vi "Reset.vi"(8 "error in (no error)":errorcluster, 11 "ChromaPowerSupply in":refnum<class "ChromaPowerSupply.lvclass">) -> (0 "error out":errorcluster, 3 "ChromaPowerSupply out":refnum<class "ChromaPowerSupply.lvclass">)   [LabVIEW 2018, in "AcPwrPlugins.lvlib" / "ChromaPowerSupply.lvclass"]
doc: "This VI resets the instrument(s) into a know state."
uses:
  ChromaPowerSupply.lvclass
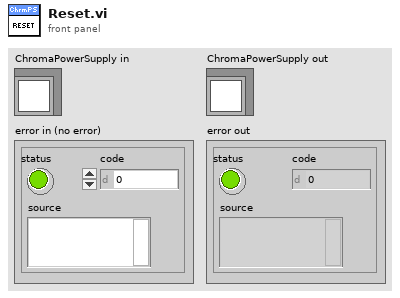
[diagram p1: front panel]
types:
  T1 = typedef "AcPwrPlugins.lvlib/ChromaPowerSupply.lvclass/Device(s)Settings.ctl" = cluster{"Phases":cluster{"Handle":string, "Instrument Options":string, "id query (T)":bool, "reset device (T)":bool, "Timing":cluster{"TimingOn":enum16{""}, "Hours":u32, "Minutes":u32, "Seconds":dbl, "CutoffVoltage":dbl}, "Connected":bool, "Output Mode":enum16{"Voltage (DC)", "Current (DC)"}, "Voltage":dbl, "Current":dbl, "Voltage Limit":dbl, "Current Limit":dbl}[], "MeasName":string}
  T2 = cluster{"Handle":string, "Instrument Options":string, "id query (T)":bool, "reset device (T)":bool, "Timing":cluster{"TimingOn":enum16{""}, "Hours":u32, "Minutes":u32, "Seconds":dbl, "CutoffVoltage":dbl}, "Connected":bool, "Output Mode":enum16{"Voltage (DC)", "Current (DC)"}, "Voltage":dbl, "Current":dbl, "Voltage Limit":dbl, "Current Limit":dbl}[]
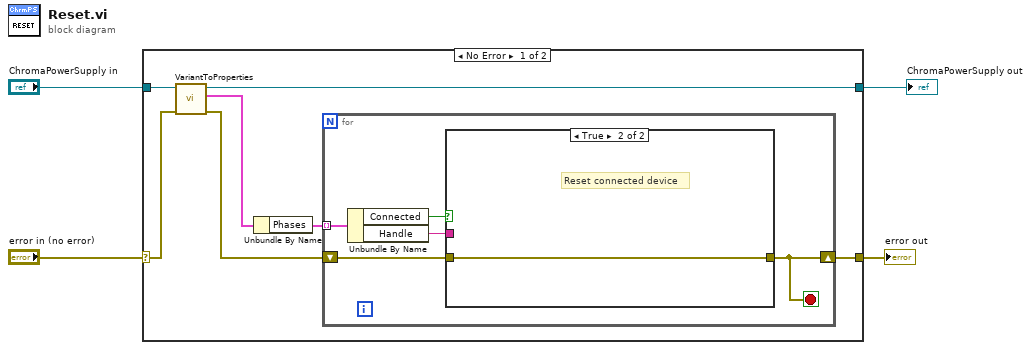
[diagram p0: block diagram]
diagram:
  n1 = case shown="No Error" "error in (no error)" {
    selector: "error in (no error)" -> [w8 w20]
    tunnel: [w11 w20] -> w1
    tunnel: [w10 w19] -> w2
    tunnel: "ChromaPowerSupply in" -> [w9 w19]
    frame No Error {
      n2 = call-dynamic "VariantToProperties.vi"("error in (no error)"=w8, "ChromaPowerSupply in"=w9) -> ("error out"=w7:errorcluster, "Device Settings"=w6:T1, "ChromaPowerSupply out"=w10:refnum<class "ChromaPowerSupply.lvclass">)  [unwired: 5 in, 2 out]
      n3 = Unbundle By Name(w6) -> ("Phases"=w5:T2)
      n4 = for {
        tunnel: w5 -> [w16] mode=indexing
        shift-right: [w13] -> w11
        shift-left: w7 -> [w15]
        stop <- w13 stop-if-true
        n5 = Unbundle By Name(w16) -> ("Connected"=w12:bool, "Handle"=w14:string)
        n6 = case shown="True" w12 {
          tunnel: w15 -> [w17 w18]
          tunnel: w14 -> [_ _]
          tunnel: [w17 w18] -> w13
          frame False {
          }
          frame True {
            # "Reset connected device"
          }
        }
      }
    }
    frame Error {
    }
  }
  "error out" <- w1
  "ChromaPowerSupply out" <- w2
